vi "RunTimeMenu_Initialize_TCE.vi"(11 "Menu in":refnum<k9>) -> (0 "files":string[](array[string]), 3 "paths":path[](array[path]))   [LabVIEW 2020]
uses:
  a2aa5e15-ca40-4839-88f0-bbf66ff86cff.vi
  96004bec-fd17-4972-871d-ca5e9cc0281a.vi
  2479bbb3-f647-4402-a6ab-e7a78c17a9d0.vi
  <vilib>/Utility/file.llb/Read Delimited Spreadsheet (string).vi
  <vilib>/Utility/file.llb/Write Delimited Spreadsheet (string).vi
  <vilib>/regexp/Match Regular Expression.xnode
panel:
  out "error out 2":errorcluster
  out "subarray":string[](array[string])
  out "error out":errorcluster
  out "Array":string[](array[string])
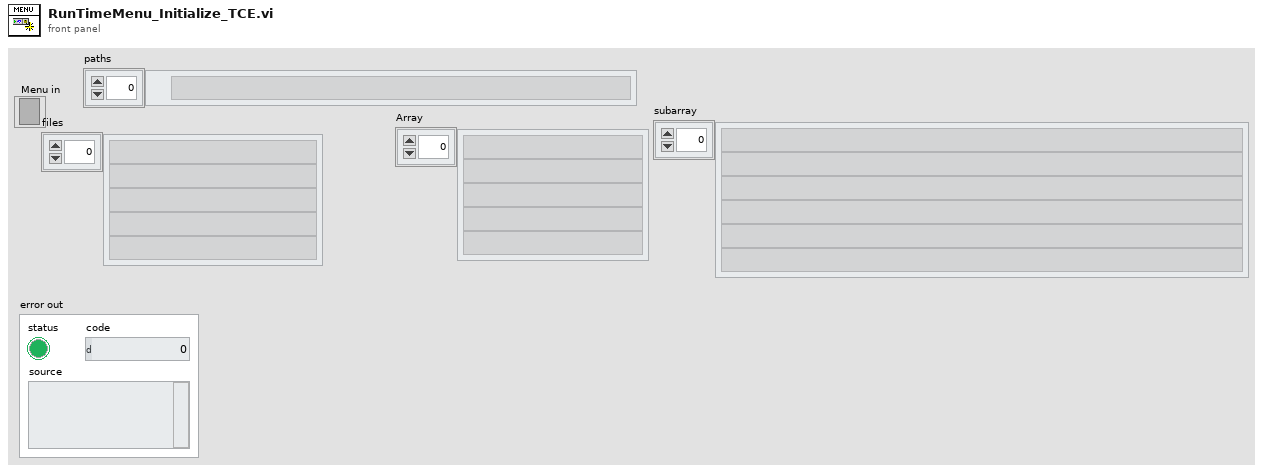
[diagram p1: front panel]
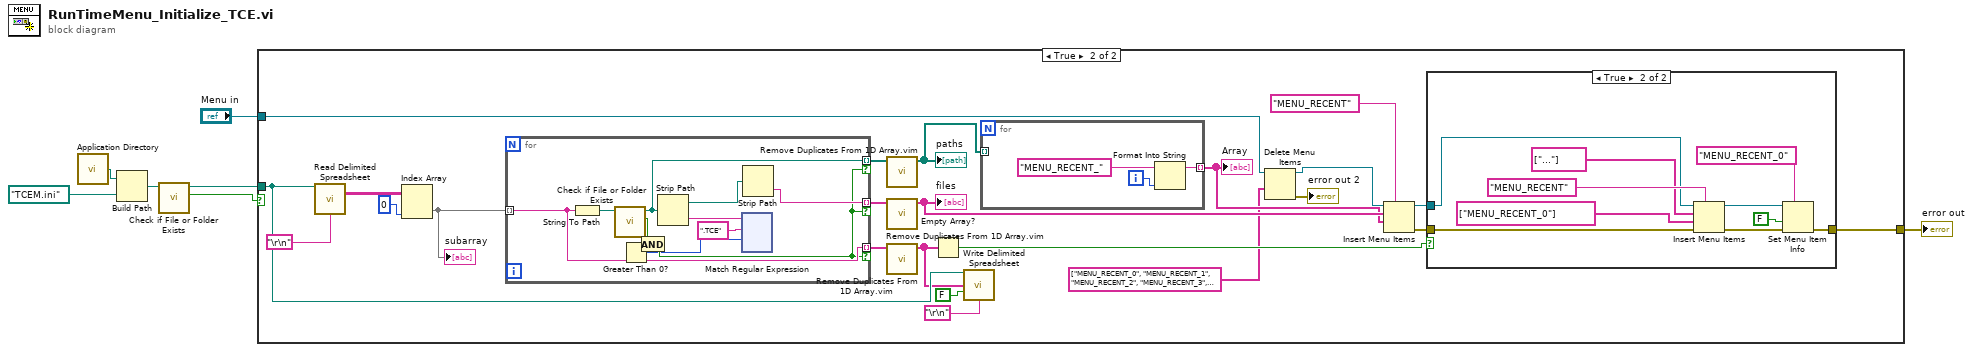
[diagram p0: block diagram]
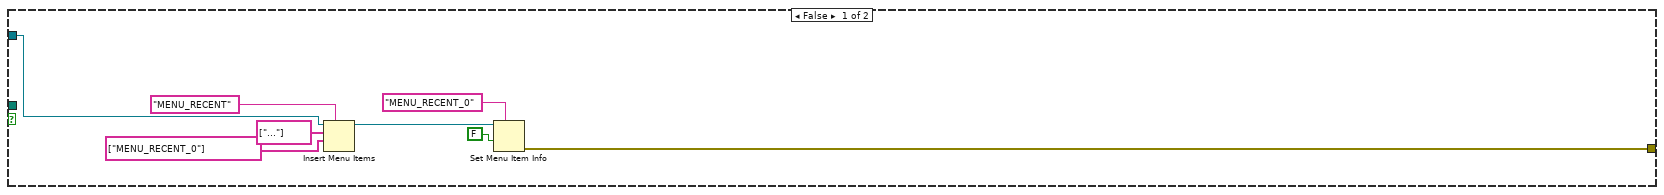
[diagram p2: hidden frame]
diagram:
  n1 = call <vilib>:"Application Directory.vi"() -> ("Application Directory"=w7:path)
  n2 = Build Path(base path=w7, name or relative path=path "TCEM.ini") -> (appended path=w5:path)
  n3 = call <vilib>:"Check if File or Folder Exists.vi"("path"=w5) -> ("file or folder exists?"=w4:bool, "dup path"=w3:path)  [unwired: 8 in, 1 out]
  n4 = case shown="True" w4 {
    tunnel: w3 -> [_ w37]
    tunnel: "Menu in" -> [w15 w20]
    tunnel: [w8 w33] -> w1
    frame False {
      n5 = Insert Menu Items(5:"MENU_RECENT" ("menu tag"), 7:string[] ["MENU_RECENT_0"] ("item tags"), 8:string[] ["..."] ("item names"), 9:w15) -> (3:w12:refnum<k9>)  [unwired: 2 in, 2 out]
      n6 = Set Menu Item Info(7:"MENU_RECENT_0" ("item tag"), 9:FALSE ("enabled"), 11:w12) -> (0:w8:errorcluster)  [unwired: 4 in, 1 out]
    }
    frame True {
      n7 = call-poly <vilib>:"Read Delimited Spreadsheet.vi"("file path (dialog if empty)"=w37, "delimiter (\\t)"="\r\n") -> ("all rows"=w32:string[][])  [unwired: 8 in, 5 out]
      n8 = Index Array(array=w32, index (col)=0 ("disabled index (col)")) -> (element=w31:string[])  [unwired: 1 in]
      "subarray" <- w31
      n9 = for {
        tunnel: w31 -> [w57] mode=indexing
        tunnel: [w62] -> w23 mode=indexing if=w55
        tunnel: [w56] -> w25 mode=indexing if=w55
        tunnel: [w57] -> w27 mode=indexing if=w55
        n10 = String To Path(string=w57) -> (path=w63:path)
        n11 = call <vilib>:"Check if File or Folder Exists.vi"("path"=w63) -> ("file or folder exists?"=w60:bool, "dup path"=w62:path)  [unwired: 8 in, 1 out]
        n12 = Strip Path(path=w62) -> (stripped path=w61:path, name=w59:string)
        n13 = xnode "Match Regular Expression"("input string"=w59, "regular expression"=".TCE") -> ("offset past match"=w54:i32)  [unwired: 4 in, 4 out]
        n14 = Greater Than 0?(x=w54) -> (x > 0?=w53:bool)
        n15 = And(x=w60, y=w53) -> (x .and. y?=w55:bool)
        n16 = Strip Path(path=w61) -> (name=w56:string)  [unwired: 1 out]
      }
      n17 = call "Remove Duplicates From 1D Array.vim"("array"=w23) -> ("array with duplicates removed"=w22:path[])  [unwired: 10 in]
      "paths" <- w22
      n18 = call "Remove Duplicates From 1D Array.vim"("array"=w25) -> ("array with duplicates removed"=w24:string[])  [unwired: 10 in]
      "files" <- w24
      n19 = call "Remove Duplicates From 1D Array.vim"("array"=w27) -> ("array with duplicates removed"=w26:string[])  [unwired: 10 in]
      n20 = Empty Array?(array=w26) -> (empty?=w35:bool)
      n21 = call-poly <vilib>:"Write Delimited Spreadsheet.vi"("file path (dialog if empty)"=w37, "1D data"=w26, "append to file? (new file:F)"=FALSE, "delimiter (\\t)"="\r\n") -> ()  [unwired: 10 in, 2 out]
      n22 = for {
        tunnel: w22 -> [_] mode=indexing
        tunnel: [w39] -> w21 mode=indexing
        i -> [w40]
        n23 = Format Into String(initial string="MENU_RECENT_", w40) -> (resulting string=w39:string)  [unwired: 2 in, 1 out]
      }
      "Array" <- w21
      n24 = Delete Menu Items(7:string[] ["MENU_RECENT_0", "MENU_RECENT_1", "MENU_RECENT_2", "MENU_RECENT_3", "MENU_RECENT_4"], 9:w20) -> (0:→"error out 2":errorcluster, 3:w19:refnum<k9>)  [unwired: 2 in]
      n25 = Insert Menu Items(5:"MENU_RECENT" ("menu tag"), 7:w21, 8:w24, 9:w19) -> (0:w34:errorcluster, 3:w18:refnum<k9>)  [unwired: 2 in, 1 out]
      n26 = case shown="True" w35 {
        tunnel: w18 -> [_ w46]
        tunnel: w34 -> [w42 w44]
        tunnel: [w42 w45] -> w33
        frame False {
        }
        frame True {
          n27 = Insert Menu Items(5:"MENU_RECENT" ("menu tag"), 6:w44, 7:string[] ["MENU_RECENT_0"] ("item tags"), 8:string[] ["..."] ("item names"), 9:w46) -> (0:w43:errorcluster, 3:w52:refnum<k9>)  [unwired: 1 in, 1 out]
          n28 = Set Menu Item Info(7:"MENU_RECENT_0" ("item tag"), 8:w43, 9:FALSE ("enabled"), 11:w52) -> (0:w45:errorcluster)  [unwired: 3 in, 1 out]
        }
      }
    }
  }
  "error out" <- w1
